vi "_TangoAttributeConfigEventHandler.vi"(3 "error in":errorcluster, 4 "timeout (ms)":i32=1000, 5 "attribute config event ref":T2) -> (0 "error out":errorcluster, 1 "attribute info":T1, 2 "event timeout":bool)   [LabVIEW 2014, in "tango.lvlib"]
uses:
  tango.lvlib
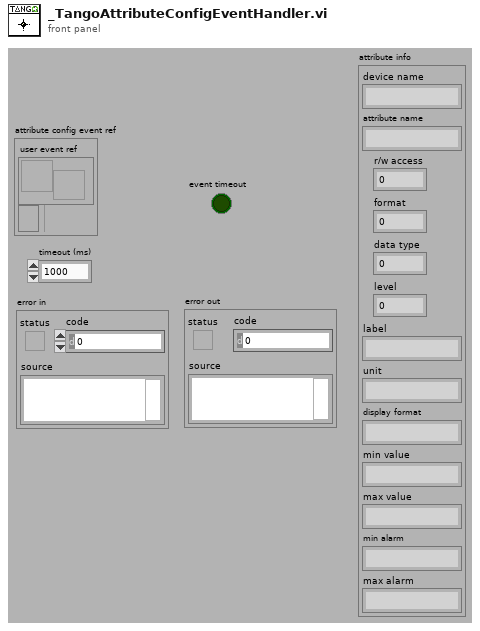
[diagram p1: front panel]
types:
  T1 = cluster{"device name":string, "attribute name":string, "r/w access":i16, "format":i16, "data type":i16, "level":i16, "label":string, "unit":string, "display format":string, "min value":string, "max value":string, "min alarm":string, "max alarm":string}
  T2 = cluster{"user event ref":refnum<user-event>, "user event reg refnum":refnum<event-registration>}
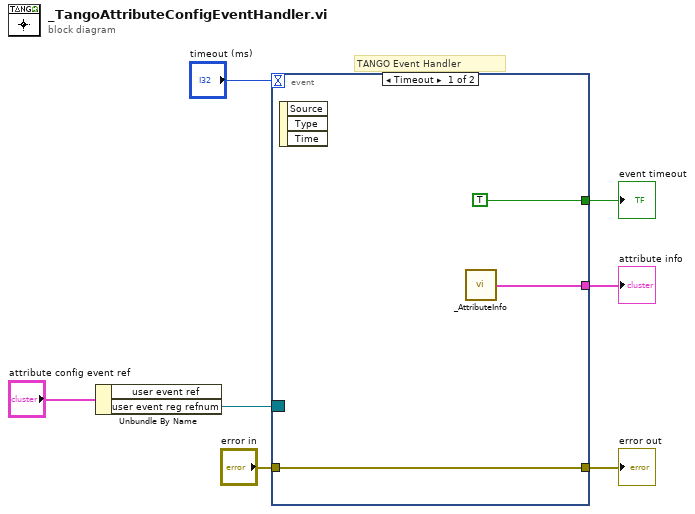
[diagram p0: block diagram]
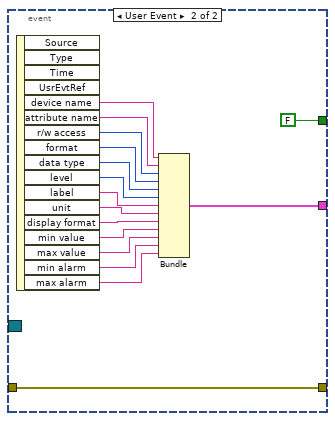
[diagram p2: hidden frame]
diagram:
  # "TANGO Event Handler"
  n1 = Unbundle By Name("attribute config event ref") -> ("user event reg refnum"=w3:refnum<event-registration>)  [unwired: 1 out]
  n2 = event shown="[0] Timeout" {
    selector: w3 -> [_ _]
    dyn-events: _ -> [_ _]
    timeout: "timeout (ms)" -> [_ _]
    tunnel: [TRUE FALSE] -> w7
    tunnel: "error in" -> [w9 w13]
    tunnel: [w9 w13] -> w5
    tunnel: [w8 w12] -> w2
    event Timeout {
      n3 = event-data() -> ()  [unwired: 1 in, 3 out]
      n4 = call "_AttributeInfo.vi"() -> ("attribute info"=w8:T1)  [unwired: 15 in]
    }
    event User Event {
      n5 = event-data() -> ("device name"=w26:string, "attribute name"=w25:string, "r/w access"=w24:i16, "format"=w23:i16, "data type"=w22:i16, "level"=w21:i16, "label"=w20:string, "unit"=w19:string, "display format"=w18:string, "min value"=w17:string, "max value"=w16:string, "min alarm"=w15:string, "max alarm"=w14:string)  [unwired: 1 in, 4 out]
      n6 = Bundle("device name"=w26, "attribute name"=w25, "r/w access"=w24, "format"=w23, "data type"=w22, "level"=w21, "label"=w20, "unit"=w19, "display format"=w18, "min value"=w17, "max value"=w16, "min alarm"=w15, "max alarm"=w14) -> (w12:T1)  [unwired: 1 in]
    }
  }
  "event timeout" <- w7
  "error out" <- w5
  "attribute info" <- w2
